vi "CallVi.vi"() -> ()   [LabVIEW 2018]
panel:
  out "VI Path":path
  out "selected path":path
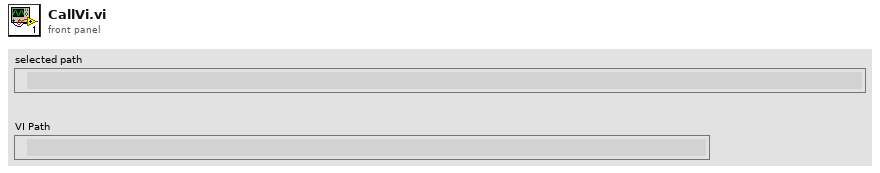
[diagram p1: front panel]
types:
  T1 = enum32{"Invalid", "Standard", "Closed", "Hidden", "Minimized", "Maximized"}
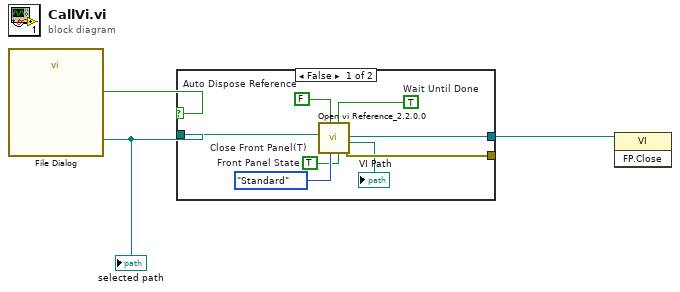
[diagram p0: block diagram]
diagram:
  n1 = call "File Dialog"() -> ("selected path"=w3:path, "cancelled"=w2:bool)  [unwired: 12 in, 2 out]
  "selected path" <- w3
  n2 = case shown="False" w2 {
    tunnel: w3 -> [w11 _]
    tunnel: [w7 _] -> _
    tunnel: [w5 _] -> w1
    frame False {
      w6 = TRUE  # Close Front Panel(T)
      w8 = T1."Standard"  # Front Panel State
      w9 = TRUE  # Wait Until Done
      w10 = FALSE  # Auto Dispose Reference
      n3 = call "Open vi Reference_2.2.0.0.vi"("Close Front Panel(T)"=w6, "Wait Until Done"=w9, "Front Panel State"=w8, "Auto Dispose Reference"=w10, "vi path"=w11) -> ("error out"=w7:errorcluster, "VI Path"=→"VI Path":path, "vi reference"=w5:refnum<vi>)  [unwired: 3 in, 1 out]
    }
    frame True {
    }
  }
  n4 = invoke class="VI" method="FP.Close"(reference=w1) -> ()  [unwired: 2 in, 3 out]
